vi "Auto_Measurement.vi"() -> ()   [LabVIEW 2018]
panel:
  in  "Dimensions":T1(ring)
  in  "Thickness (nm)":string="50"
  in  "Email on completion?":bool
  in  "Email recipient":string="rgiri@uw.edu"
  in  "Subject":string="OECT Scans Done"
  in  "Message":string="Hi Raj"
  out "Current Scan #":dbl
  out "Current V_G":dbl
  in  "Transfer Curve Controls":T2={"V_G Start"=-0.85, "V_G Finish"=0.0, "V_G Step Size"=0.025, "Software Averages"=5, "Delay between \naverages (ms)"=200.0, "Preread delay (ms)"=5000.0, "First bias settle (ms)"=2000.0, "V_DS"=-0.6, "Current Compliance\nLimit 237 (A)"=0.1, "Keithley 237 GPIB address"="17", "Current Compliance\nLimit (A) Ke2400"=1.0, "VISA resource name "="GPIB0::24::INSTR", "Number of Transfer Curves"=1.0, "Voltage Compliance Limit 237 (V)"=10.0} {"Voltage Compliance Limit 237 (V)" format="%#.3f"; "Current Compliance\nLimit (A) Ke2400" format="%#.3e"; "Current Compliance\nLimit 237 (A)" format="%#.3f"; "V_DS" format="%#_13g"; "First bias settle (ms)" format="%#.2f"; "Preread delay (ms)" format="%.2f"; "Delay between \naverages (ms)" format="%#.3f"; "V_G Step Size" format="%#.3g"; "V_G Finish" format="%#.3g"; "V_G Start" format="%#.3g"}
  in  "Output Curve Controls":T3={"V_DS Start"=-0.7, "V_DS Finish"=0.0, "V_DS Step Size"=0.1, "Software Averages"=5, "Delay between \naverages (ms)"=200.0, "Preread delay (ms)"=5000.0, "First bias settle (ms)"=2000.0, "Current Compliance\nLimit 237 (A)"=0.1, "Keithley 237 GPIB address"="17", "Current Compliance\nLimit (A) Ke2400"=1.0, "VISA resource name "="GPIB0::24::INSTR", "Voltage Compliance Limit 237 (V)"=10.0, "V_G Array"=[-0.5, -0.8]} {"Voltage Compliance Limit 237 (V)" format="%#.3f"; "Current Compliance\nLimit (A) Ke2400" format="%#.3e"; "Current Compliance\nLimit 237 (A)" format="%#.3f"; "First bias settle (ms)" format="%#.2f"; "Preread delay (ms)" format="%.2f"; "Delay between \naverages (ms)" format="%#.3f"; "V_DS Step Size" format="%#.3g"; "V_DS Finish" format="%#.3g"; "V_DS Start" format="%#.3g"}
  # "Output Curve Display"
  # "Transfer Curve Display"
  # "Scan Settings"
  # "Keithley 237 (V_DS) Settings"
  # "Keithley 2400 (V_G) Settings"
  # "Scan Settings"
  # "Keithley 237 (V_DS) Settings"
  # "Keithley 2400 (V_G) Settings"
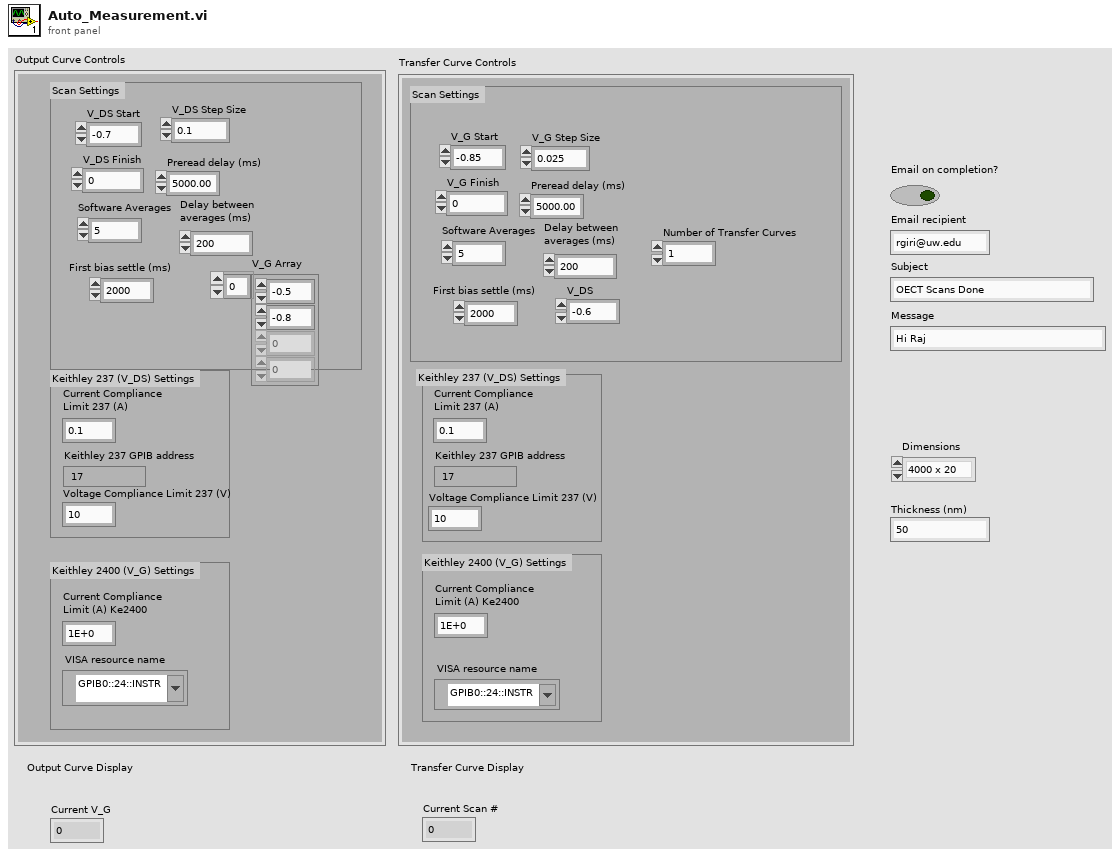
[diagram p1: front panel]
types:
  T1 = enum16{"4000 x 20", "2000 x 20", "1000 x 20", "800 x 20", "400 x 20", "200 x 20", "100 x 20"}
  T2 = cluster{"V_G Start":dbl, "V_G Finish":dbl, "V_G Step Size":dbl, "Software Averages":i16, "Delay between \naverages (ms)":dbl, "Preread delay (ms)":dbl, "First bias settle (ms)":dbl, "V_DS":dbl, "Current Compliance\nLimit 237 (A)":dbl, "Keithley 237 GPIB address":string, "Current Compliance\nLimit (A) Ke2400":dbl, "VISA resource name ":refnum<visa-resource-name>, "Number of Transfer Curves":dbl, "Voltage Compliance Limit 237 (V)":dbl}
  T3 = cluster{"V_DS Start":dbl, "V_DS Finish":dbl, "V_DS Step Size":dbl, "Software Averages":i16, "Delay between \naverages (ms)":dbl, "Preread delay (ms)":dbl, "First bias settle (ms)":dbl, "Current Compliance\nLimit 237 (A)":dbl, "Keithley 237 GPIB address":string, "Current Compliance\nLimit (A) Ke2400":dbl, "VISA resource name ":refnum<visa-resource-name>, "Voltage Compliance Limit 237 (V)":dbl, "V_G Array":dbl[]}
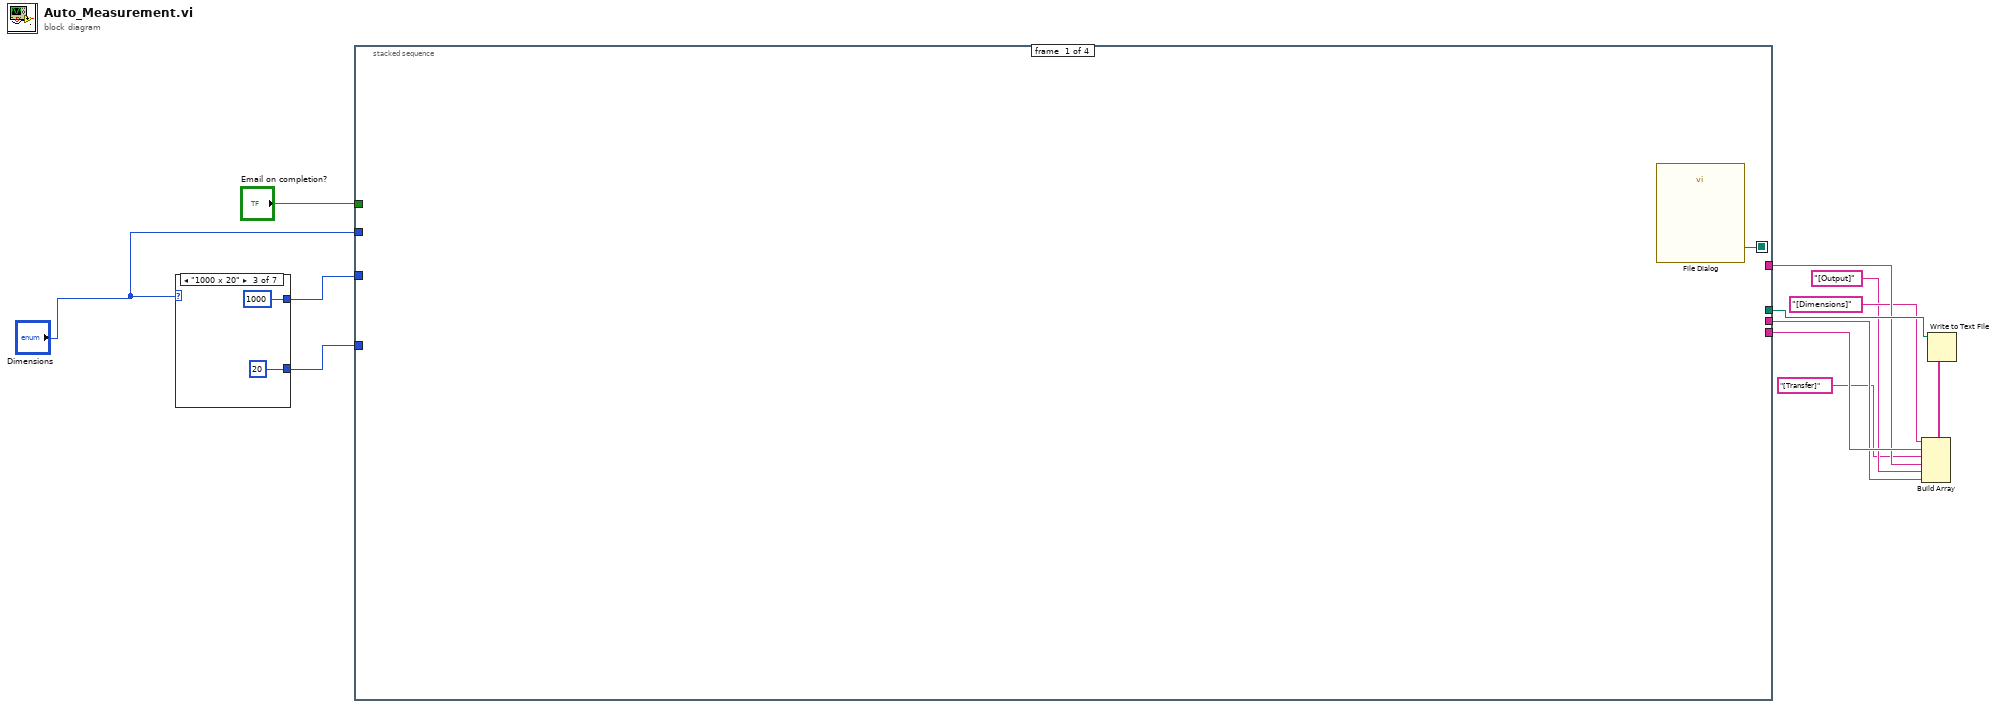
[diagram p0: block diagram]
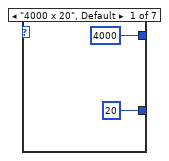
[diagram p2: hidden frame]
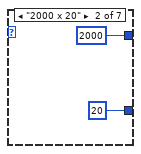
[diagram p3: hidden frame]
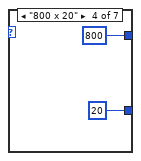
[diagram p4: hidden frame]
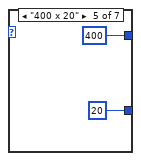
[diagram p5: hidden frame]
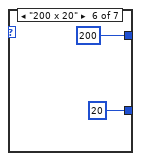
[diagram p6: hidden frame]
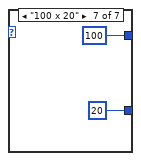
[diagram p7: hidden frame]
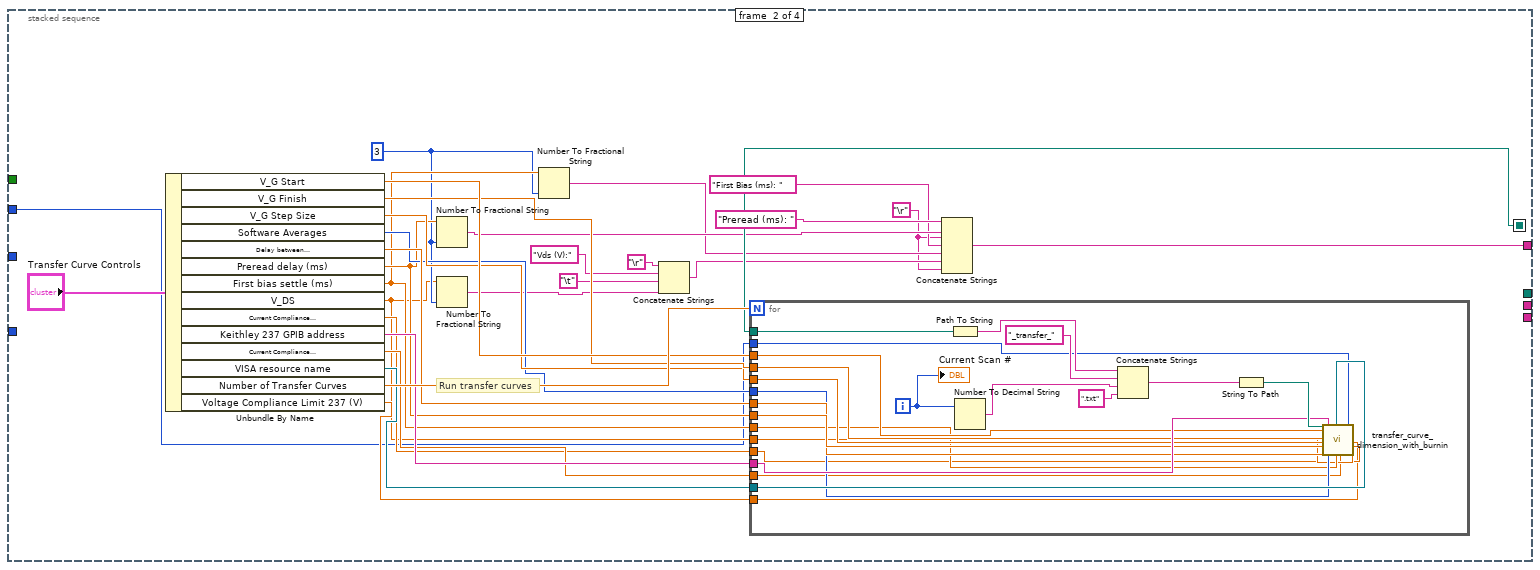
[diagram p8: hidden frame]
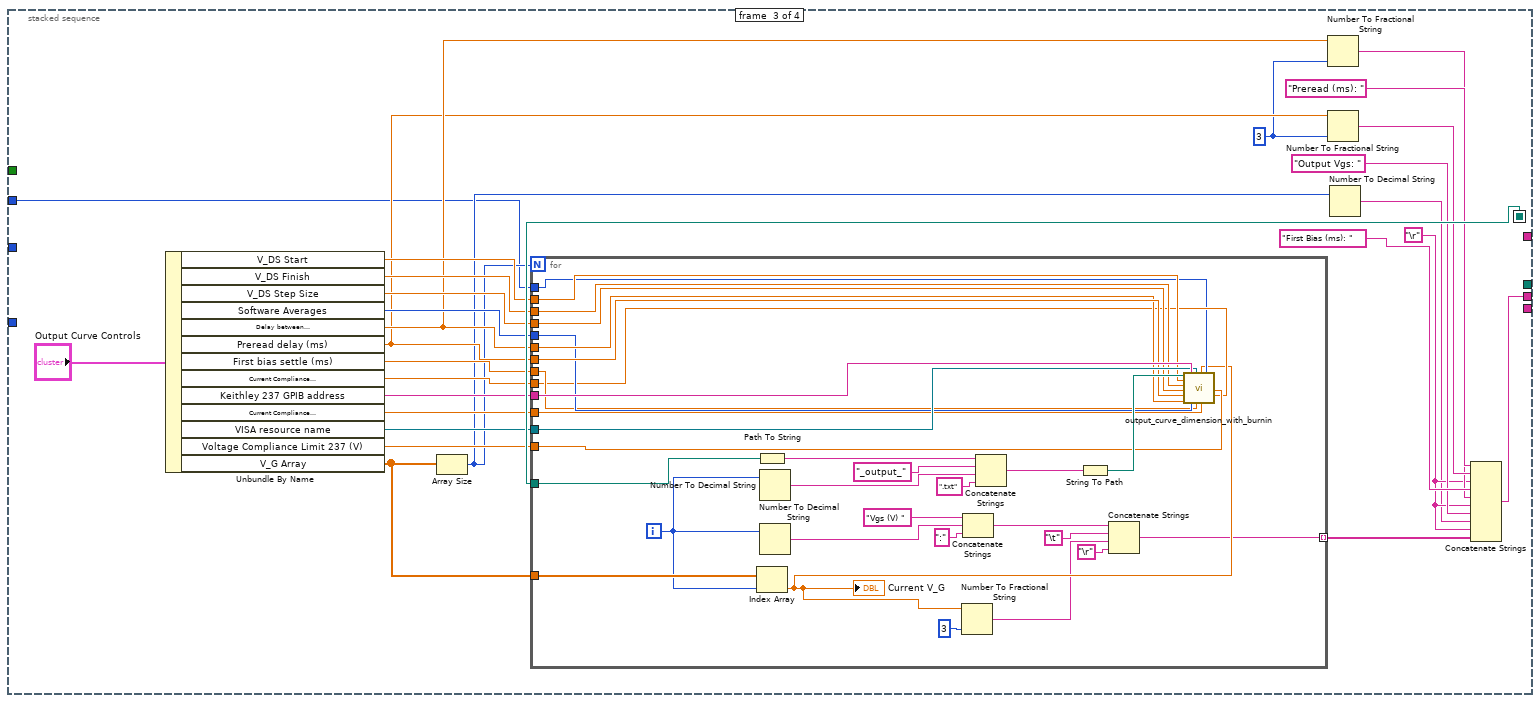
[diagram p9: hidden frame]
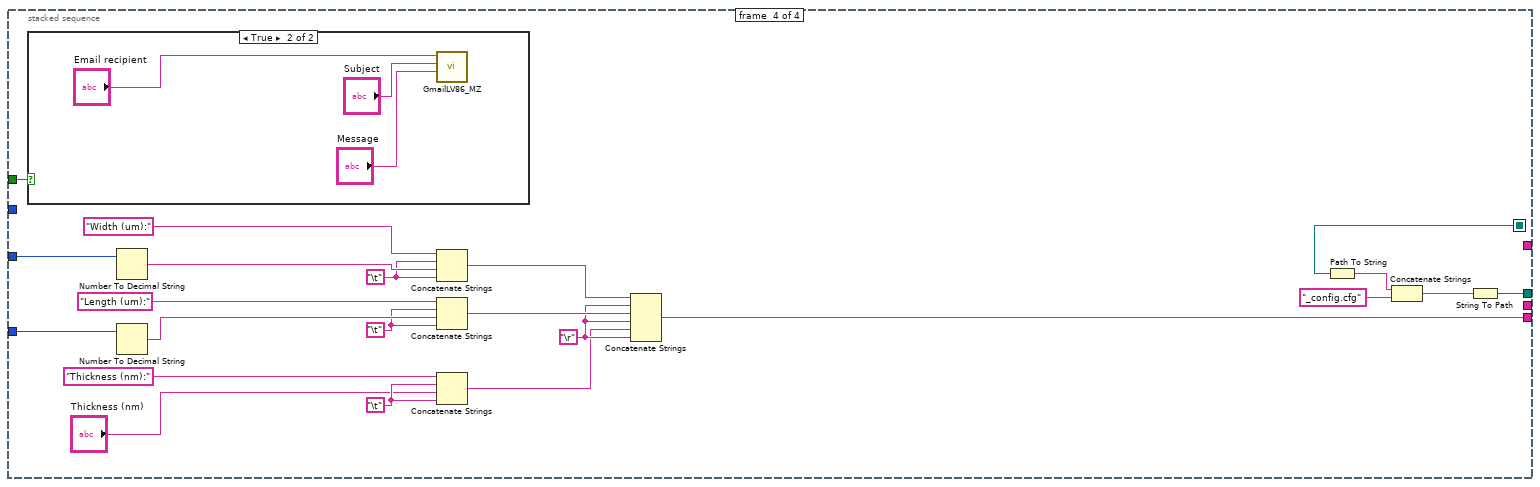
[diagram p10: hidden frame]
diagram:
  n1 = case shown="\"1000 x 20\"" "Dimensions" {
    tunnel: [4000 2000 1000 800 400 200 100] -> w3
    tunnel: [20 20 20 20 20 20 20] -> w2
    frame "4000 x 20", Default {
    }
    frame "2000 x 20" {
    }
    frame "1000 x 20" {
    }
    frame "800 x 20" {
    }
    frame "400 x 20" {
    }
    frame "200 x 20" {
    }
    frame "100 x 20" {
    }
  }
  n2 = stacked-sequence {
    seq-local: [w27 _ _ _] -> [_ w54 w104 w158]
    tunnel: "Email on completion?" -> [_ _ _ w159]
    tunnel: [_ w37 _ _] -> w8
    tunnel: [_ _ w86 _] -> w7
    tunnel: [_ _ _ w148] -> w11
    tunnel: [_ _ _ w145] -> w9
    tunnel: w3 -> [_ _ _ w139]
    tunnel: w2 -> [_ _ _ w138]
    tunnel: "Dimensions" -> [_ w28 w79 _]
    frame #0 {
      n3 = call "File Dialog"() -> ("selected path"=w27:path)  [unwired: 12 in, 3 out]
    }
    frame #1 {
      w35 = 3
      w29 = "\r"
      # "Run transfer curves"
      n4 = Unbundle By Name("Transfer Curve Controls") -> ("V_G Start"=w51:dbl, "V_G Finish"=w50:dbl, "V_G Step Size"=w49:dbl, "Software Averages"=w47:i16, "Delay between \naverages (ms)"=w48:dbl, "Preread delay (ms)"=w43:dbl, "First bias settle (ms)"=w42:dbl, "V_DS"=w34:dbl, "Current Compliance\nLimit 237 (A)"=w45:dbl, "Keithley 237 GPIB address"=w53:string, "Current Compliance\nLimit (A) Ke2400"=w46:dbl, "VISA resource name"=w52:refnum<visa-resource-name>, "Number of Transfer Curves"=w55:dbl, "Voltage Compliance Limit 237 (V)"=w44:dbl)
      n5 = Number To Fractional String(number=w43, precision (6)=w35) -> (F-format string=w40:string)  [unwired: 2 in]
      n6 = Number To Fractional String(number=w34, precision (6)=w35) -> (F-format string=w32:string)  [unwired: 2 in]
      n7 = Number To Fractional String(number=w42, precision (6)=w35) -> (F-format string=w38:string)  [unwired: 2 in]
      n8 = Concatenate Strings("\r", "Vds (V):", "\t", w32) -> (w31:string)
      n9 = for {
        N: w55 -> [_]
        tunnel: w54 -> [w78]
        tunnel: w53 -> [w74]
        tunnel: w52 -> [w73]
        tunnel: w51 -> [w72]
        tunnel: w50 -> [w71]
        tunnel: w49 -> [w70]
        tunnel: w43 -> [w69]
        tunnel: w48 -> [w68]
        tunnel: w47 -> [w67]
        tunnel: w42 -> [w66]
        tunnel: w34 -> [w65]
        tunnel: w46 -> [w64]
        tunnel: w45 -> [w63]
        tunnel: w44 -> [w62]
        tunnel: w28 -> [w57]
        i -> [w58]
        n10 = Path To String(path=w78) -> (string=w77:string)
        n11 = Number To Decimal String(number=w58) -> (decimal integer string=w60:string)  [unwired: 1 in]
        n12 = Concatenate Strings(w77, "_transfer_", w60, ".txt") -> (w76:string)
        n13 = String To Path(string=w76) -> (path=w75:path)
        n14 = call "transfer_curve_dimension_with_burnin.vi"("File Path"=w75, "V_G Start"=w72, "V_G Finish"=w71, "V_G Step Size"=w70, "Preread delay (ms)"=w69, "Delay between \naverages (ms)"=w68, "Keithley 237 GPIB address"=w74, "Software Averages"=w67, "VISA resource name"=w73, "First bias settle (ms)"=w66, "Current Compliance\nLimit (A) Ke2400"=w64, "Dimensions"=w57, "Voltage Compliance Limit 237 (V)"=w62, "Current Compliance\nLimit 237 (A)"=w63, "V_DS"=w65) -> ()  [unwired: 13 in]
        "Current Scan #" <- w58
      }
      n15 = Concatenate Strings("Preread (ms): ", w40, w29, "First Bias (ms): ", w38, w31, w29) -> (w37:string)
    }
    frame #2 {
      w82 = "\r"
      w83 = 3
      n16 = Unbundle By Name("Output Curve Controls") -> ("V_DS Start"=w101:dbl, "V_DS Finish"=w100:dbl, "V_DS Step Size"=w99:dbl, "Software Averages"=w98:i16, "Delay between \naverages (ms)"=w93:dbl, "Preread delay (ms)"=w92:dbl, "First bias settle (ms)"=w97:dbl, "Current Compliance\nLimit 237 (A)"=w94:dbl, "Keithley 237 GPIB address"=w103:string, "Current Compliance\nLimit (A) Ke2400"=w96:dbl, "VISA resource name"=w102:refnum<visa-resource-name>, "Voltage Compliance Limit 237 (V)"=w95:dbl, "V_G Array"=w91:dbl[])
      n17 = Array Size(array=w91) -> (size(s)=w81:i32)
      n18 = for {
        N: w81 -> [_]
        tunnel: w91 -> [w137]
        tunnel: w104 -> [w136]
        tunnel: w103 -> [w130]
        tunnel: w102 -> [w129]
        tunnel: w101 -> [w127]
        tunnel: w100 -> [w126]
        tunnel: w99 -> [w125]
        tunnel: w92 -> [w124]
        tunnel: w93 -> [w123]
        tunnel: w98 -> [w122]
        tunnel: w97 -> [w121]
        tunnel: w96 -> [w120]
        tunnel: w95 -> [w119]
        tunnel: w94 -> [w118]
        tunnel: w79 -> [w117]
        tunnel: [w113] -> w84 mode=indexing
        i -> [w110]
        n19 = Path To String(path=w136) -> (string=w135:string)
        n20 = Index Array(array=w137, index=w110) -> (element=w116:dbl)
        "Current V_G" <- w116
        n21 = Number To Decimal String(number=w110) -> (decimal integer string=w133:string)  [unwired: 1 in]
        n22 = Number To Decimal String(number=w110) -> (decimal integer string=w107:string)  [unwired: 1 in]
        n23 = Number To Fractional String(number=w116, precision (6)=3) -> (F-format string=w115:string)  [unwired: 2 in]
        n24 = Concatenate Strings("Vgs (V) ", w107, ":") -> (w108:string)
        n25 = Concatenate Strings(w135, "_output_", w133, ".txt") -> (w131:string)
        n26 = String To Path(string=w131) -> (path=w128:path)
        n27 = Concatenate Strings(w108, "\t", w115, "\r") -> (w113:string)
        n28 = call "output_curve_dimension_with_burnin.vi"("File Path"=w128, "V_DS Start"=w127, "V_DS Finish"=w126, "V_DS Step Size"=w125, "Preread delay (ms)"=w124, "Delay between \naverages (ms)"=w123, "Keithley 237 GPIB address"=w130, "Software Averages"=w122, "VISA resource name"=w129, "First bias settle (ms)"=w121, "V_G"=w116, "Current Compliance\nLimit (A) Ke2400"=w120, "Dimensions"=w117, "Voltage Compliance Limit 237 (V)"=w119, "Current Compliance\nLimit 237 (A)"=w118) -> ()  [unwired: 5 in]
      }
      n29 = Number To Fractional String(number=w93, precision (6)=w83) -> (F-format string=w87:string)  [unwired: 2 in]
      n30 = Number To Fractional String(number=w92, precision (6)=w83) -> (F-format string=w89:string)  [unwired: 2 in]
      n31 = Number To Decimal String(number=w81) -> (decimal integer string=w80:string)  [unwired: 1 in]
      n32 = Concatenate Strings("Preread (ms): ", w89, w82, "First Bias (ms): ", w87, w82, "Output Vgs: ", w80, w82, w84) -> (w86:string)
    }
    frame #3 {
      w141 = "\t"
      w144 = "\r"
      w149 = "\t"
      w152 = "\t"
      n33 = case shown="True" w159 {
        frame False {
        }
        frame True {
          n34 = call "GmailLV86_MZ.vi"("Body"="Message", "Subject"="Subject", "Recipient's Email Address"="Email recipient") -> ()  [unwired: 7 in]
        }
      }
      n35 = Number To Decimal String(number=w139) -> (decimal integer string=w154:string)  [unwired: 1 in]
      n36 = Number To Decimal String(number=w138) -> (decimal integer string=w151:string)  [unwired: 1 in]
      n37 = Concatenate Strings("Width (um):", w152, w154, w152) -> (w147:string)
      n38 = Concatenate Strings("Length (um):", w149, w151, w149) -> (w146:string)
      n39 = Concatenate Strings("Thickness (nm):", w141, "Thickness (nm)", w141) -> (w143:string)
      n40 = Concatenate Strings(w147, w144, w146, w144, w143, w144) -> (w145:string)
      n41 = Path To String(path=w158) -> (string=w157:string)
      n42 = Concatenate Strings(w157, "_config.cfg") -> (w155:string)
      n43 = String To Path(string=w155) -> (path=w148:path)
    }
  }
  n44 = Build Array("[Dimensions]", w9, "[Transfer]", w8, "[Output]", w7) -> (w10:string[])
  n45 = Write to Text File(file (use dialog)=w11, text=w10) -> ()  [unwired: 2 in, 3 out]
